vi "Start button.vi"(8 "error in (no error)":errorcluster, 11 "VISA resource name":refnum<visa-resource-name>) -> (0 "error out":errorcluster, 3 "VISA resource name out":refnum<visa-resource-name>)   [LabVIEW 2017, in "SR400.lvlib"]
doc: "Sending the CS command has the same effect as\npressing the START key. The CS command may\nbe sent at any time but only has an effect if the\ncounters are paused or in reset. If the DWELL TIME is EXTERNAL, the CS command will start\na count period. A CH command may be sent to\nterminate the count period."
uses:
  SR400.lvlib
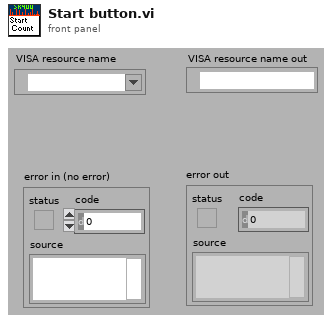
[diagram p1: front panel]
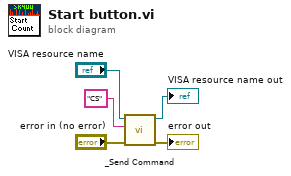
[diagram p0: block diagram]
diagram:
  n1 = call "_Send Command.vi"("error in (no error)"="error in (no error)", "Command"="CS" ("command"), "VISA resource name"="VISA resource name") -> ("error out"=→"error out":errorcluster, "VISA resource name out"=→"VISA resource name out":refnum<visa-resource-name>)  [unwired: 1 in, 6 out]
